vi "Validation Class.vi"() -> ()   [LabVIEW 2020, in "Library Instrument & Equipement.lvlib" / "Library FireBase.lvlib" / "Firebase Scan.lvclass"]
uses:
  Firebase Scan.lvclass
  C:/Users/ngarcin/OneDrive - Altyor/Standard TB/Class/Firebase/Source/Firebase Altyor/Firebase Altyor.lvclass
  C:/Users/ngarcin/OneDrive - Altyor/Standard TB/Class/Firebase/Source/Firebase Driver/Firebase Driver.lvclass
  Firebase Scan.lvclass/Firebase Scan.ctl
panel:
  out "Get_Data_With_Condition":T1(array[cluster])
  out "Get_Sub_Collection":T2(array[cluster])
  out "tableau ajouté":T3(array[cluster])
  out "Get_Data":T3(array[cluster])
  out "sortie d'erreur":errorcluster
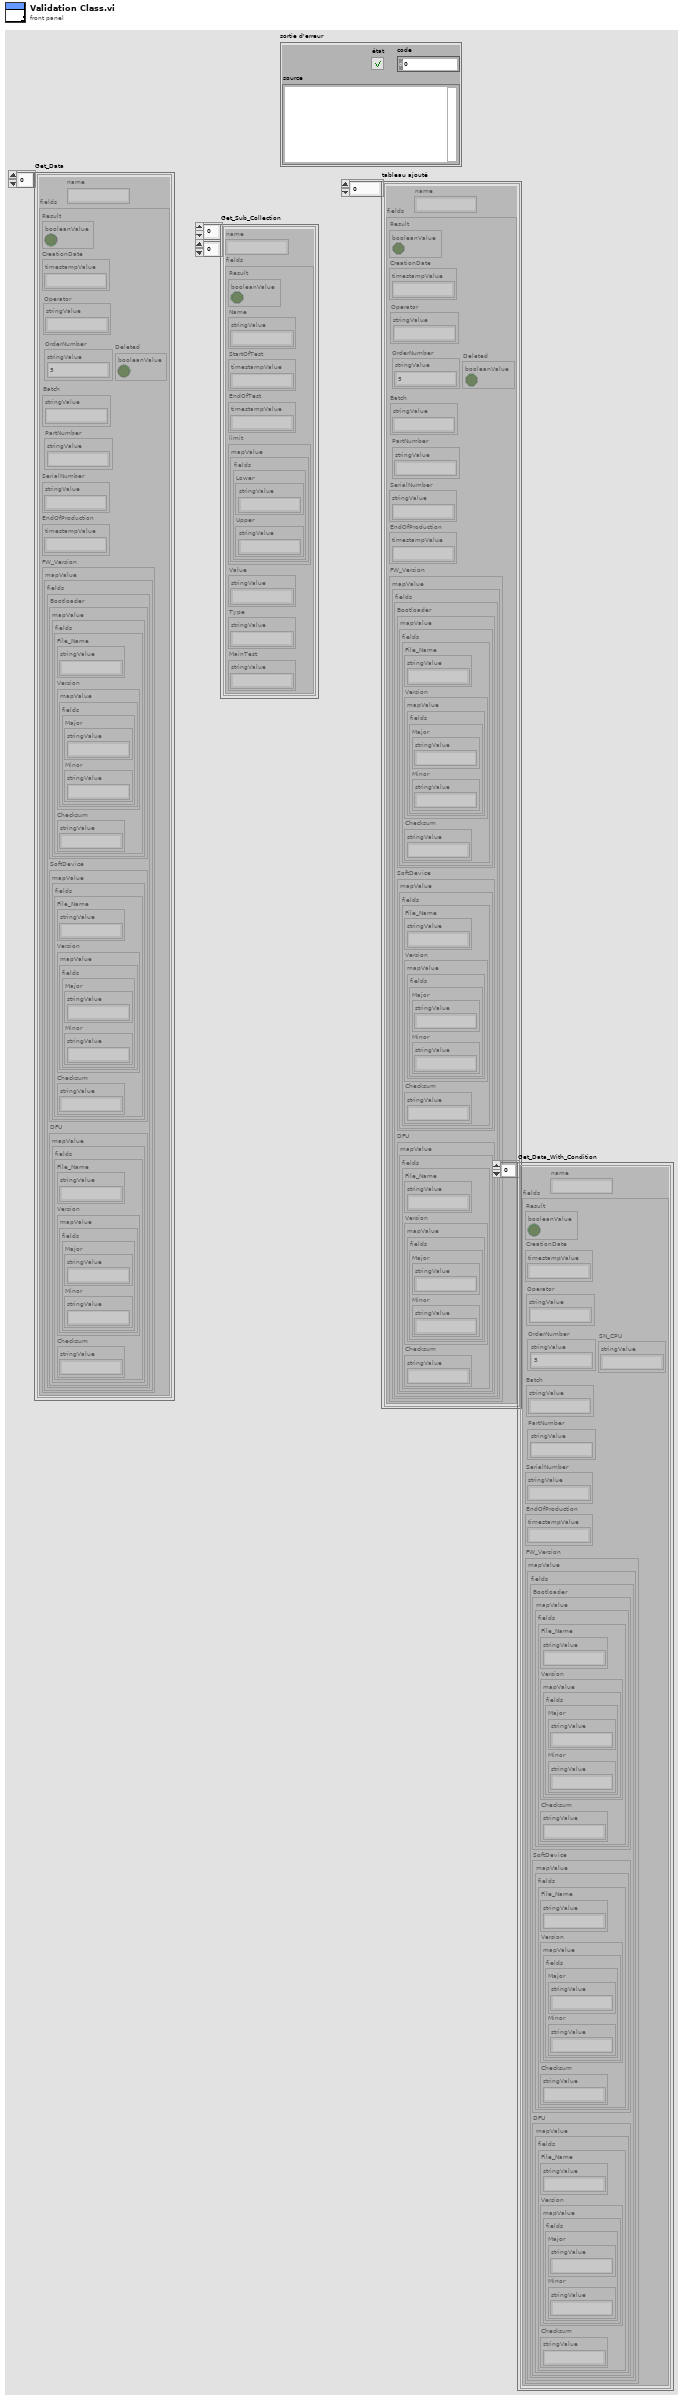
[diagram p1: front panel]
types:
  T1 = cluster{"name":string, "fields":cluster{"Result":cluster{"booleanValue":bool}, "CreationDate":cluster{"timestampValue":string}, "Batch":cluster{"stringValue":string}, "SerialNumber":cluster{"stringValue":string}, "EndOfProduction":cluster{"timestampValue":string}, "FW_Version":cluster{"mapValue":cluster{"fields":cluster{"Bootloader":cluster{"mapValue":cluster{"fields":cluster{"File_Name":cluster{"stringValue":string}, "Version":cluster{"mapValue":cluster{"fields":cluster{"Major":cluster{"stringValue":string}, "Minor":cluster{"stringValue":string}}}}, "Checksum":cluster{"stringValue":string}}}}, "SoftDevice":cluster{"mapValue":cluster{"fields":cluster{"File_Name":cluster{"stringValue":string}, "Version":cluster{"mapValue":cluster{"fields":cluster{"Major":cluster{"stringValue":string}, "Minor":cluster{"stringValue":string}}}}, "Checksum":cluster{"stringValue":string}}}}, "DFU":cluster{"mapValue":cluster{"fields":cluster{"File_Name":cluster{"stringValue":string}, "Version":cluster{"mapValue":cluster{"fields":cluster{"Major":cluster{"stringValue":string}, "Minor":cluster{"stringValue":string}}}}, "Checksum":cluster{"stringValue":string}}}}}}}, "PartNumber":cluster{"stringValue":string}, "OrderNumber":cluster{"stringValue":string}, "Operator":cluster{"stringValue":string}, "SN_CPU":cluster{"stringValue":string}}}[]
  T2 = cluster{"name":string, "fields":cluster{"Result":cluster{"booleanValue":bool}, "Name":cluster{"stringValue":string}, "StartOfTest":cluster{"timestampValue":string}, "EndOfTest":cluster{"timestampValue":string}, "limit":cluster{"mapValue":cluster{"fields":cluster{"Lower":cluster{"stringValue":string}, "Upper":cluster{"stringValue":string}}}}, "Value":cluster{"stringValue":string}, "Type":cluster{"stringValue":string}, "MainTest":cluster{"stringValue":string}}}[][]
  T3 = cluster{"name":string, "fields":cluster{"Result":cluster{"booleanValue":bool}, "CreationDate":cluster{"timestampValue":string}, "Batch":cluster{"stringValue":string}, "SerialNumber":cluster{"stringValue":string}, "EndOfProduction":cluster{"timestampValue":string}, "FW_Version":cluster{"mapValue":cluster{"fields":cluster{"Bootloader":cluster{"mapValue":cluster{"fields":cluster{"File_Name":cluster{"stringValue":string}, "Version":cluster{"mapValue":cluster{"fields":cluster{"Major":cluster{"stringValue":string}, "Minor":cluster{"stringValue":string}}}}, "Checksum":cluster{"stringValue":string}}}}, "SoftDevice":cluster{"mapValue":cluster{"fields":cluster{"File_Name":cluster{"stringValue":string}, "Version":cluster{"mapValue":cluster{"fields":cluster{"Major":cluster{"stringValue":string}, "Minor":cluster{"stringValue":string}}}}, "Checksum":cluster{"stringValue":string}}}}, "DFU":cluster{"mapValue":cluster{"fields":cluster{"File_Name":cluster{"stringValue":string}, "Version":cluster{"mapValue":cluster{"fields":cluster{"Major":cluster{"stringValue":string}, "Minor":cluster{"stringValue":string}}}}, "Checksum":cluster{"stringValue":string}}}}}}}, "PartNumber":cluster{"stringValue":string}, "OrderNumber":cluster{"stringValue":string}, "Operator":cluster{"stringValue":string}, "Deleted":cluster{"booleanValue":bool}}}[]
  T4 = cluster{"Result":cluster{"booleanValue":bool}, "Name":cluster{"stringValue":string}, "StartOfTest":cluster{"timestampValue":string}, "EndOfTest":cluster{"timestampValue":string}, "limit":cluster{"mapValue":cluster{"fields":cluster{"Lower":cluster{"stringValue":string}, "Upper":cluster{"stringValue":string}}}}, "Value":cluster{"stringValue":string}, "Type":cluster{"stringValue":string}, "MainTest":cluster{"stringValue":string}}
  T5 = cluster{"Result":cluster{"booleanValue":bool}, "CreationDate":cluster{"timestampValue":string}, "Batch":cluster{"stringValue":string}, "SerialNumber":cluster{"stringValue":string}, "EndOfProduction":cluster{"timestampValue":string}, "FW_Version":cluster{"mapValue":cluster{"fields":cluster{"Bootloader":cluster{"mapValue":cluster{"fields":cluster{"File_Name":cluster{"stringValue":string}, "Version":cluster{"mapValue":cluster{"fields":cluster{"Major":cluster{"stringValue":string}, "Minor":cluster{"stringValue":string}}}}, "Checksum":cluster{"stringValue":string}}}}, "SoftDevice":cluster{"mapValue":cluster{"fields":cluster{"File_Name":cluster{"stringValue":string}, "Version":cluster{"mapValue":cluster{"fields":cluster{"Major":cluster{"stringValue":string}, "Minor":cluster{"stringValue":string}}}}, "Checksum":cluster{"stringValue":string}}}}, "DFU":cluster{"mapValue":cluster{"fields":cluster{"File_Name":cluster{"stringValue":string}, "Version":cluster{"mapValue":cluster{"fields":cluster{"Major":cluster{"stringValue":string}, "Minor":cluster{"stringValue":string}}}}, "Checksum":cluster{"stringValue":string}}}}}}}, "PartNumber":cluster{"stringValue":string}, "OrderNumber":cluster{"stringValue":string}, "Operator":cluster{"stringValue":string}, "Deleted":cluster{"booleanValue":bool}}
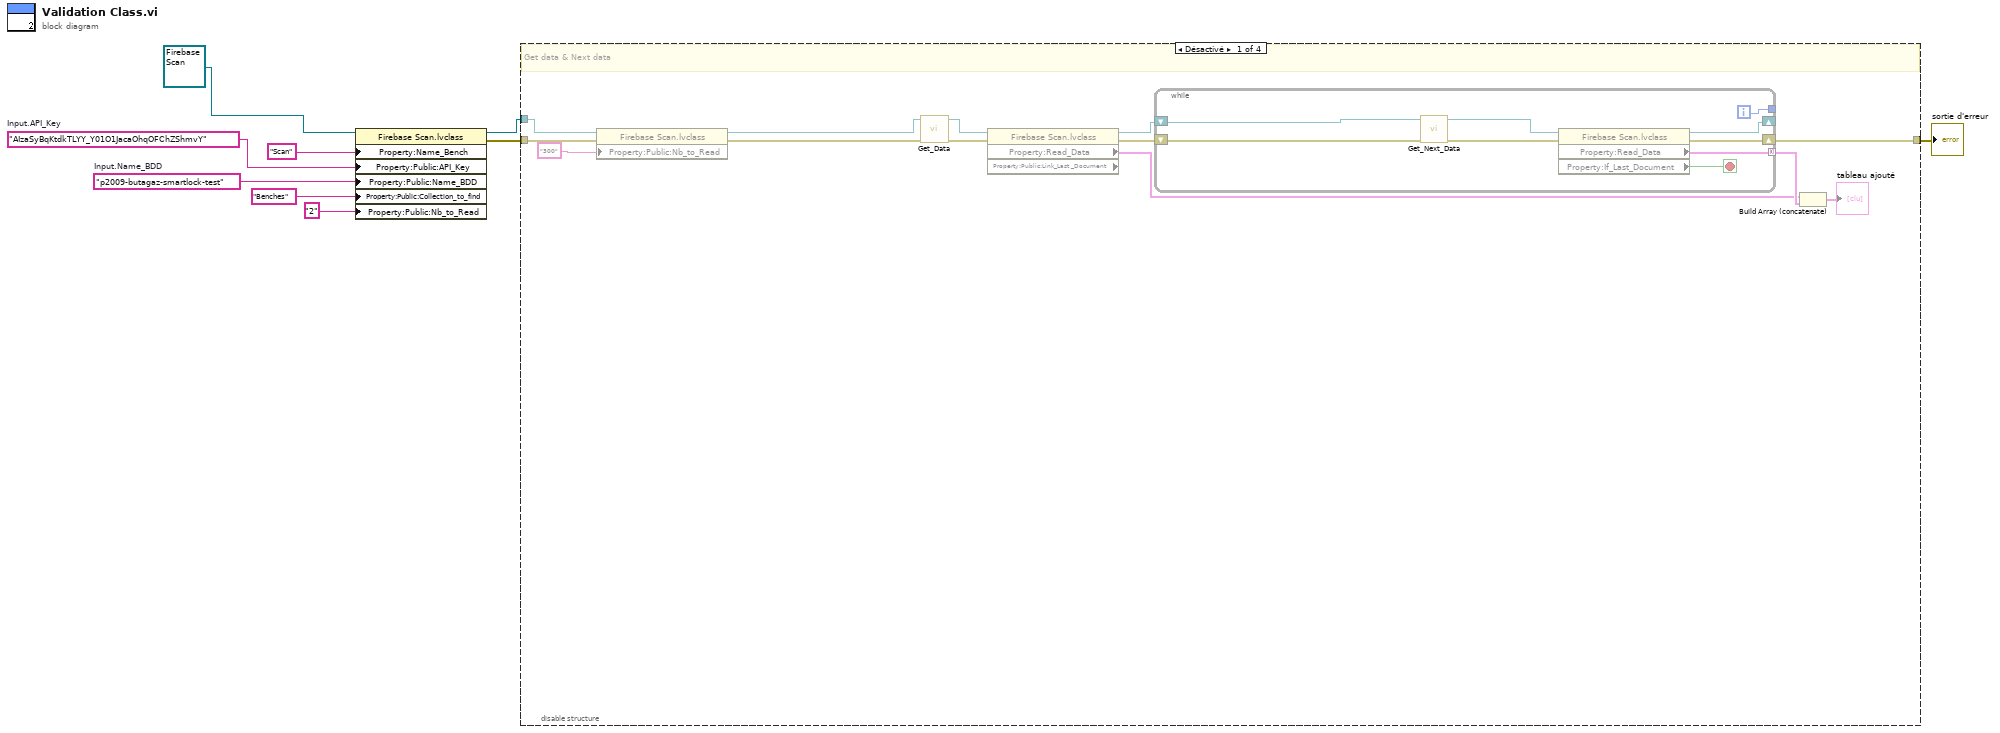
[diagram p0: block diagram]
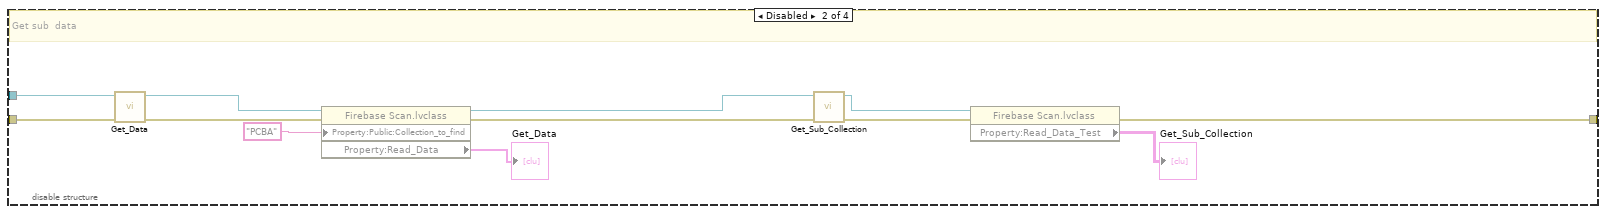
[diagram p2: hidden frame]
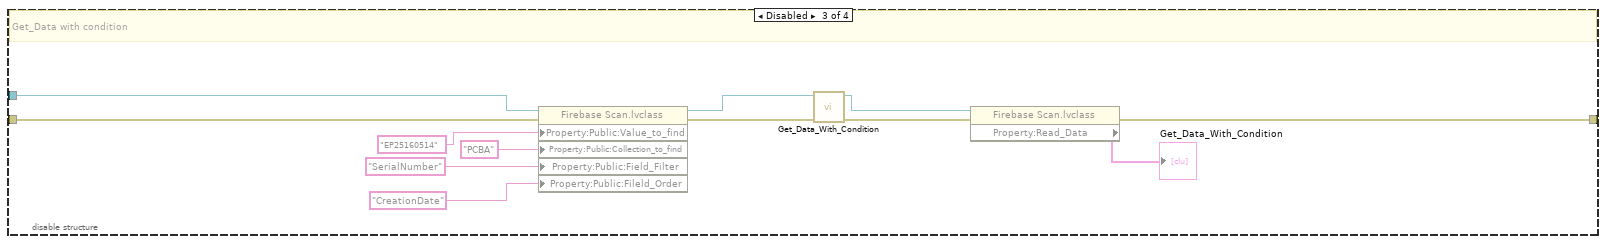
[diagram p3: hidden frame]
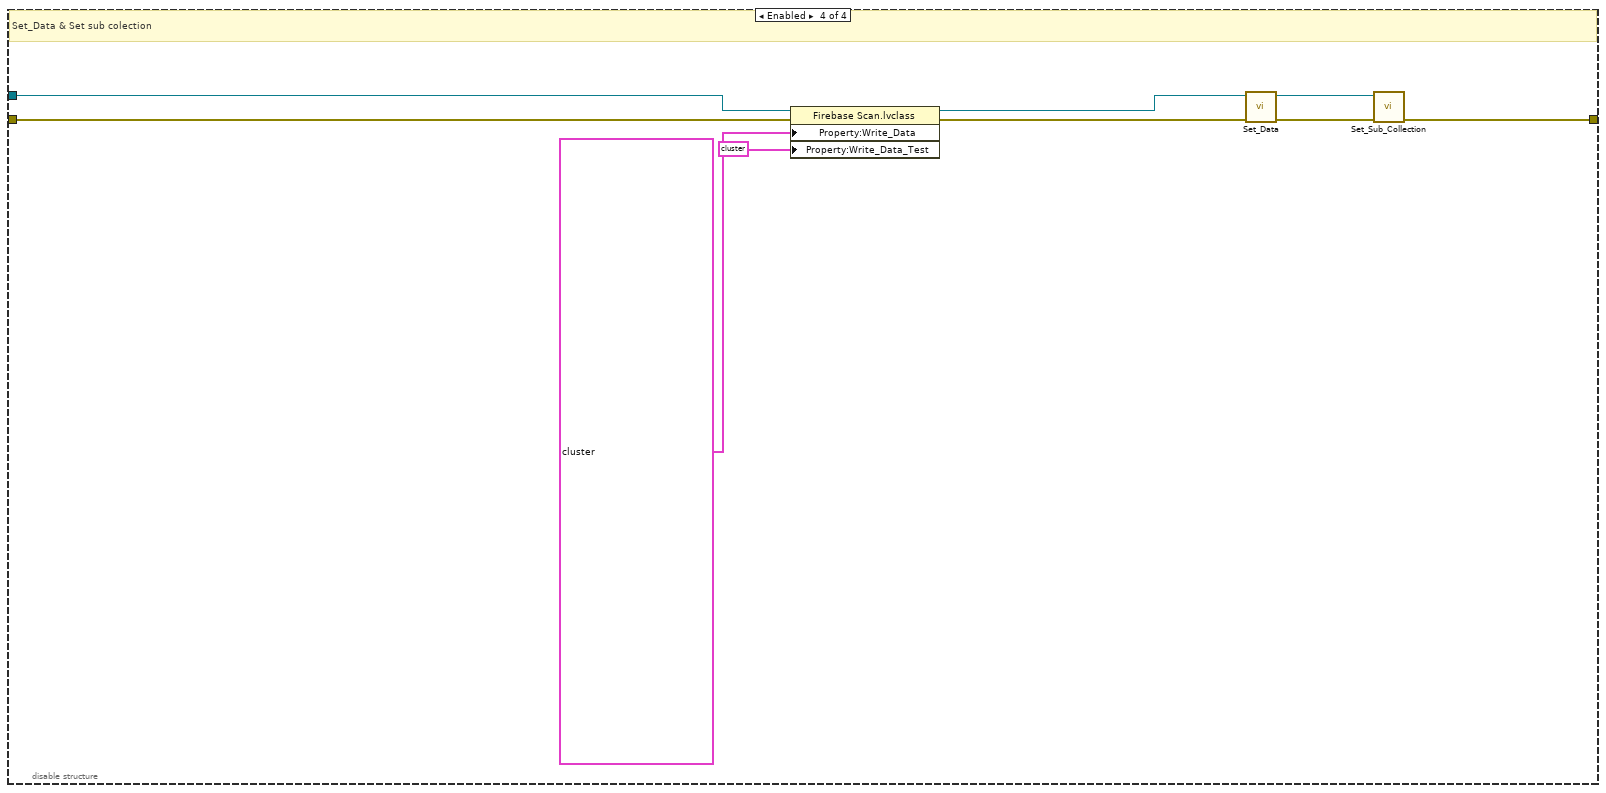
[diagram p4: hidden frame]
diagram:
  w5 = "p2009-butagaz-smartlock-test"  # Input.Name_BDD
  w6 = "AIzaSyBqKtdkTLYY_Y01O1JacaOhqOFChZShmvY"  # Input.API_Key
  n1 = property class="Firebase Scan.lvclass"(reference=refnum<class "Firebase Scan.lvclass"> refnum ("Build Library FireBase.lvlib:Firebase Scan.lvclass"), "Property:Name_Bench"="Scan" ("Set_Name_Bench"), "Property:Public:API_Key"=w6, "Property:Public:Name_BDD"=w5, "Property:Public:Collection_to_find"="Benches" ("Collection_to_find"), "Property:Public:Nb_to_Read"="2" ("Nb_to_Read")) -> (reference out=w3:refnum<class "Firebase Scan.lvclass">, error out=w4:errorcluster)  [unwired: 1 in]
  n2 = disable-structure shown="Désactivé" {
    disable-tunnel: [w22 w43 w46 w58] -> w8
    disable-tunnel: w4 -> [w12 w36 w45 w57]
    disable-tunnel: w3 -> [w14 w34 w44 w56]
    frame Disabled {
      # "Get data & Next data"
      n3 = property class="Firebase Scan.lvclass"(reference=w14, error in=w12, "Property:Public:Nb_to_Read"="300" ("Nb_to_Read")) -> (reference out=w13:refnum<class "Firebase Scan.lvclass">, error out=w11:errorcluster)
      n4 = call-dynamic "Get_Data.vi"("error in (no error)"=w11, "Firebase Benches en entrée"=w13) -> ("error out"=w19:errorcluster, "Firebase Benches en sortie"=w18:refnum<class "Firebase Scan.lvclass">)  [unwired: 8 in]
      n5 = property class="Firebase Scan.lvclass" props=["Property:Read_Data", "Property:Public:Link_Last _Document"](reference=w18, error in=w19) -> (reference out=w17:refnum<class "Firebase Scan.lvclass">, error out=w16:errorcluster, "Property:Read_Data"=w15:T3)  [unwired: 1 out]
      n6 = while {
        shift-right: [w31] -> w22
        shift-left: w16 -> [w24]
        tunnel: [w28] -> w21 mode=concatenating
        shift-right: [w30] -> _
        shift-left: w17 -> [w26]
        tunnel: [w29] -> _
        i -> [w29]
        stop <- w27 stop-if-true
        n7 = call-dynamic "Get_Next_Data.vi"("error in (no error)"=w24, "Firebase Benches en entrée"=w26) -> ("error out"=w23:errorcluster, "Firebase Benches en sortie"=w25:refnum<class "Firebase Scan.lvclass">)  [unwired: 8 in]
        n8 = property class="Firebase Scan.lvclass"(reference=w25, error in=w23) -> (reference out=w30:refnum<class "Firebase Scan.lvclass">, error out=w31:errorcluster, "Property:Read_Data"=w28:T3, "Property:If_Last_Document"=w27:bool)
      }
      n9 = Build Array (concatenate)(w15, w21) -> (→"tableau ajouté":T3)
    }
    frame Disabled {
      # "Get sub  data"
      n10 = call-dynamic "Get_Data.vi"("error in (no error)"=w36, "Firebase Benches en entrée"=w34) -> ("error out"=w35:errorcluster, "Firebase Benches en sortie"=w33:refnum<class "Firebase Scan.lvclass">)  [unwired: 8 in]
      n11 = property class="Firebase Scan.lvclass"(reference=w33, error in=w35, "Property:Public:Collection_to_find"="PCBA" ("Set_Name_Bench")) -> (reference out=w40:refnum<class "Firebase Scan.lvclass">, error out=w39:errorcluster, "Property:Read_Data"=→"Get_Data":T3)
      n12 = call-dynamic "Get_Sub_Collection.vi"("error in (no error)"=w39, "Firebase Benches en entrée"=w40) -> ("error out"=w38:errorcluster, "Firebase Benches en sortie"=w37:refnum<class "Firebase Scan.lvclass">)  [unwired: 8 in]
      n13 = property class="Firebase Scan.lvclass"(reference=w37, error in=w38) -> (error out=w43:errorcluster, "Property:Read_Data_Test"=→"Get_Sub_Collection":T2)  [unwired: 1 out]
    }
    frame Disabled {
      # "Get_Data with condition"
      n14 = property class="Firebase Scan.lvclass"(reference=w44, error in=w45, "Property:Public:Value_to_find"="EP25160514" ("Value_to_find"), "Property:Public:Collection_to_find"="PCBA" ("Set_Name_Bench"), "Property:Public:Field_Filter"="SerialNumber" ("Field_Filter"), "Property:Public:Fileld_Order"="CreationDate" ("Fileld_Order")) -> (reference out=w51:refnum<class "Firebase Scan.lvclass">, error out=w50:errorcluster)
      n15 = call-dynamic "Get_Data_With_Condition.vi"("error in (no error)"=w50, "Firebase Benches en entrée"=w51) -> ("error out"=w47:errorcluster, "Firebase Benches en sortie"=w49:refnum<class "Firebase Scan.lvclass">)  [unwired: 8 in]
      n16 = property class="Firebase Scan.lvclass"(reference=w49, error in=w47) -> (error out=w46:errorcluster, "Property:Read_Data"=→"Get_Data_With_Condition":T3)  [unwired: 1 out]
    }
    frame Enabled {
      # "Set_Data & Set sub colection"
      n17 = property class="Firebase Scan.lvclass"(reference=w56, error in=w57, "Property:Write_Data"=T5 {"Result"={"booleanValue"=TRUE}, "CreationDate"={"timestampValue"="2023-06-13T16:56:05.299Z"}, "Batch"={"stringValue"=""}, "SerialNumber"={"stringValue"="EP26160514"}, "EndOfProduction"={"timestampValue"="2023-06-13T16:56:05.299Z"}, "FW_Version"={"mapValue"={"fields"={"Bootloader"={"mapValue"={"fields"={"File_Name"={"stringValue"=""}, "Version"={"mapValue"={"fields"={"Major"={"stringValue"=""}, "Minor"={"stringValue"=""}}}}, "Checksum"={"stringValue"=""}}}}, "SoftDevice"={"mapValue"={"fields"={"File_Name"={"stringValue"=""}, "Version"={"mapValue"={"fields"={"Major"={"stringValue"=""}, "Minor"={"stringValue"=""}}}}, "Checksum"={"stringValue"=""}}}}, "DFU"={"mapValue"={"fields"={"File_Name"={"stringValue"=""}, "Version"={"mapValue"={"fields"={"Major"={"stringValue"=""}, "Minor"={"stringValue"=""}}}}, "Checksum"={"stringValue"=""}}}}}}}, "PartNumber"={"stringValue"="048454542"}, "OrderNumber"={"stringValue"=""}, "Operator"={"stringValue"="Nothing"}, "Deleted"={"booleanValue"=FALSE}} ("fields"), "Property:Write_Data_Test"=T4 {"Result"={"booleanValue"=TRUE}, "Name"={"stringValue"="Position"}, "StartOfTest"={"timestampValue"="2023-06-13T16:56:05.299Z"}, "EndOfTest"={"timestampValue"="2023-06-13T16:56:05.299Z"}, "limit"={"mapValue"={"fields"={"Lower"={"stringValue"=""}, "Upper"={"stringValue"=""}}}}, "Value"={"stringValue"="B10"}, "Type"={"stringValue"="String  "}, "MainTest"={"stringValue"=""}} ("fields")) -> (reference out=w62:refnum<class "Firebase Scan.lvclass">, error out=w61:errorcluster)
      n18 = call-dynamic "Set_Data.vi"("error in (no error)"=w61, "Firebase Benches en entrée"=w62) -> ("error out"=w59:errorcluster, "Firebase Benches en sortie"=w60:refnum<class "Firebase Scan.lvclass">)  [unwired: 8 in]
      n19 = call-dynamic "Set_Sub_Collection.vi"("error in (no error)"=w59, "Firebase PCBA en entrée"=w60) -> ("error out"=w58:errorcluster)  [unwired: 8 in, 1 out]
    }
  }
  "sortie d'erreur" <- w8
